vi "Level2a.vi"() -> ()   [LabVIEW 2014]
doc: "Use this template to build a standard state machine design pattern. Each state executes code and determines which state to transition to. Contrast this design pattern with the User Interface Event Handler pattern, in which code executes in response to user actions. Contrast this design pattern also with the Queued Message Handler pattern, in which each message handling code can queue zero or more new messages."
uses:
  subVIs/Level2aState.ctl
panel:
  out "Current Time":timestamp format="%<%I:%M:%S %p\n%x>T"
  out "Input Data":dbl(graph)
  in  "Timer 2 Enabled":bool
  in  "Timer 1 Enabled":bool
  in  "Stop":bool
  out "Value > 0?":bool
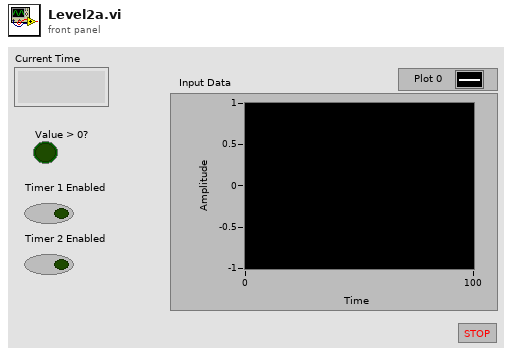
[diagram p1: front panel]
types:
  T1 = typedef "Level2aState.ctl" = enum16{"Check Inputs", "Check Clocks", "Clocks OnOff", "Generate Data", "Update Clock", "Stop"}
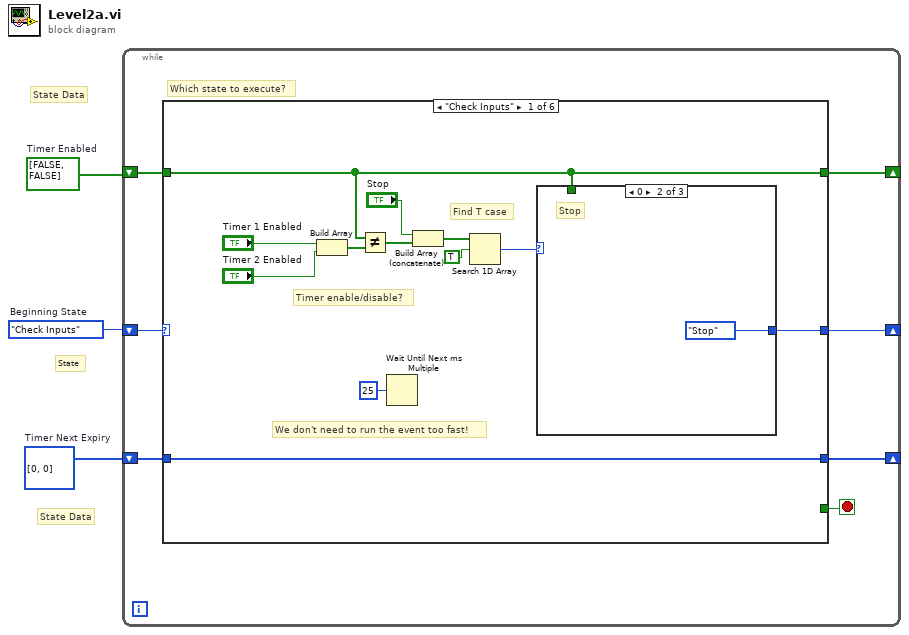
[diagram p0: block diagram]
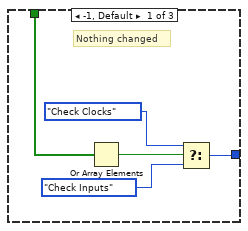
[diagram p2: hidden frame]
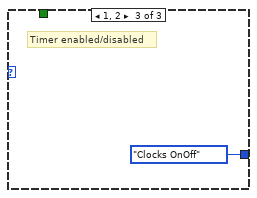
[diagram p3: hidden frame]
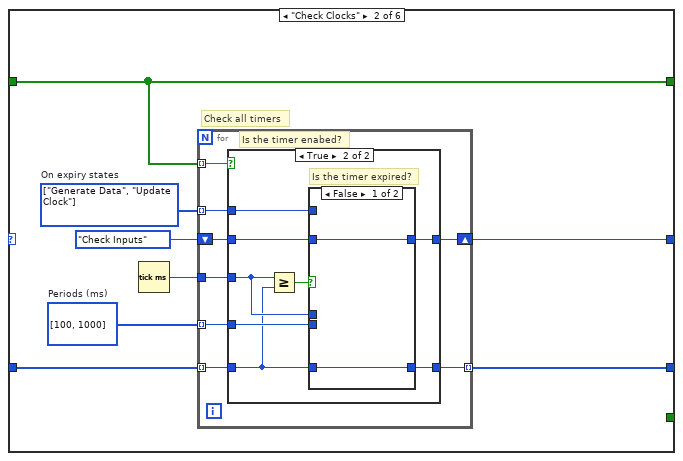
[diagram p4: hidden frame]
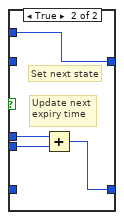
[diagram p6: hidden frame]
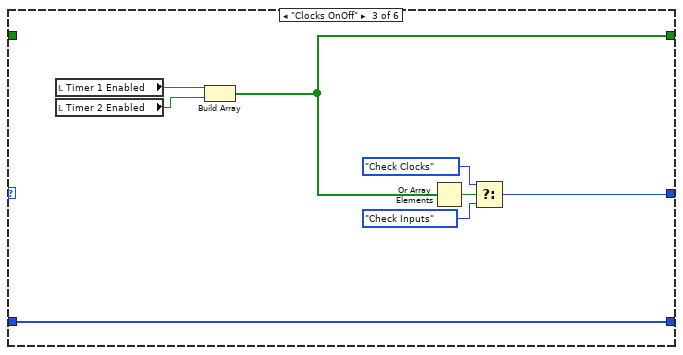
[diagram p7: hidden frame]
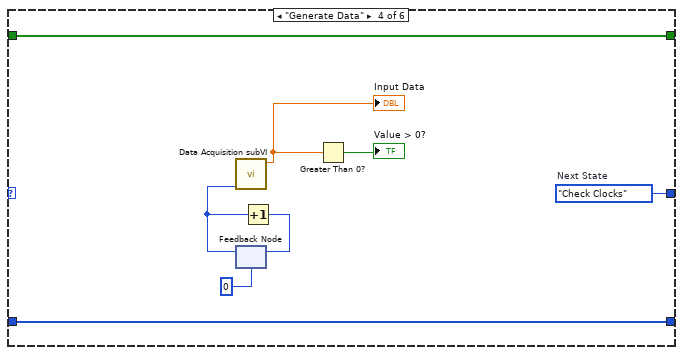
[diagram p8: hidden frame]
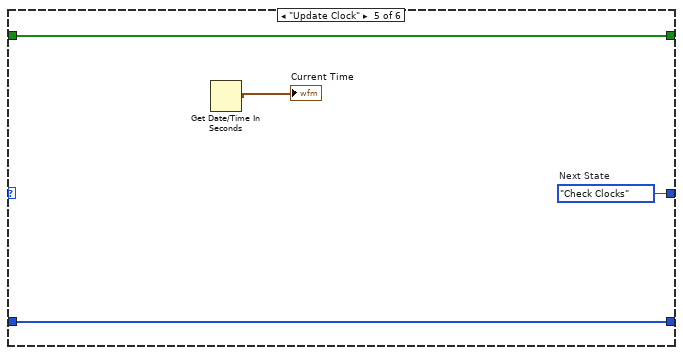
[diagram p9: hidden frame]
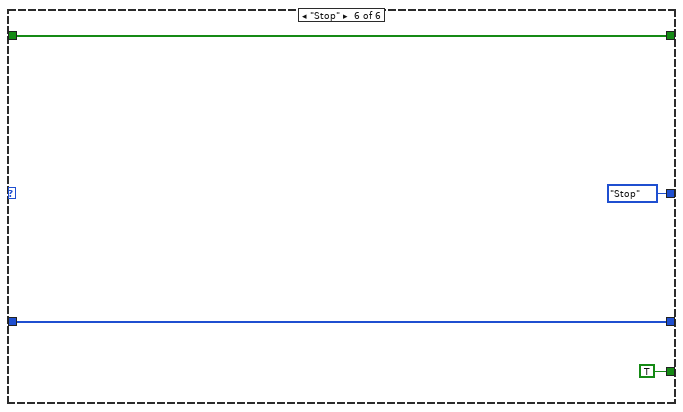
[diagram p10: hidden frame]
diagram:
  w1 = bool[] [FALSE, FALSE]  # Timer Enabled
  w2 = u32[] [0, 0]  # Timer Next Expiry
  w3 = Level2aState."Check Inputs"  # Beginning State
  # "State"
  # "State Data"
  # "State Data"
  n1 = while {
    shift-right: [w6] -> _
    shift-left: w3 -> [w9]
    shift-right: [w5] -> _
    shift-left: w2 -> [w10]
    shift-right: [w7] -> _
    shift-left: w1 -> [w8]
    stop <- w4 stop-if-true
    # "Which state to execute?"
    n2 = case shown="\"Check Inputs\"" w9 {
      tunnel: w10 -> [w12 w37 w62 w75 w80 w83]
      tunnel: w8 -> [w13 w36 _ w77 w81 w82]
      tunnel: [w13 w36 w67 w77 w81 w82] -> w7
      tunnel: [w14 w32 w63 w76 w79 Level2aState."Stop" ("Next State")] -> w6
      tunnel: [w12 w31 w62 w75 w80 w83] -> w5
      tunnel: [_ _ _ _ _ TRUE] -> w4
      frame "Check Inputs" {
        # "We don't need to run the event too fast!"
        # "Find T case"
        # "Timer enable/disable?"
        n3 = Build Array("Timer 1 Enabled", "Timer 2 Enabled") -> (w20:bool[])
        n4 = Not Equal?(x=w13, y=w20) -> (x != y?=w18:bool[])
        n5 = Wait Until Next ms Multiple(millisecond multiple=u32 25) -> ()  [unwired: 1 out]
        n6 = Build Array (concatenate)("Stop", w18) -> (w17:bool[])
        n7 = Search 1D Array(1D array=w17, element=TRUE) -> (index of element=w15:i32)  [unwired: 1 in]
        n8 = case shown="0" w15 {
          tunnel: [w23 Level2aState."Stop" ("States") Level2aState."Clocks OnOff" ("States")] -> w14
          tunnel: w13 -> [w27 _ _]
          frame -1, Default {
            # "Nothing changed"
            n9 = Or Array Elements(Boolean array=w27) -> (logical OR=w26:bool)
            n10 = Select(t=Level2aState."Check Clocks" ("States"), s=w26, f=Level2aState."Check Inputs" ("States")) -> (s? t:f=w23:T1)
          }
          frame 0 {
            # "Stop"
          }
          frame 1, 2 {
            # "Timer enabled/disabled"
          }
        }
      }
      frame "Check Clocks" {
        w33 = T1[] [enum."Generate Data", enum."Update Clock"] items=["Check Inputs", "Check Clocks", "Clocks OnOff", "Generate Data", "Update Clock", "Stop"]  # On expiry states
        w34 = u32[] [100, 1000]  # Periods (ms)
        # "Check all timers"
        n11 = Tick Count (ms)() -> (millisecond timer value=w35:u32)
        n12 = for {
          tunnel: w37 -> [w43] mode=indexing
          tunnel: w36 -> [w45] mode=indexing
          tunnel: [w44] -> w31 mode=indexing
          shift-right: [w38] -> w32
          shift-left: Level2aState."Check Inputs" -> [w42]
          tunnel: w35 -> [w41]
          tunnel: w34 -> [w40] mode=indexing
          tunnel: w33 -> [w39] mode=indexing
          # "Is the timer enabed?"
          n13 = case shown="True" w45 {
            tunnel: [w47 w52] -> w44
            tunnel: w43 -> [w47 w51]
            tunnel: w42 -> [w46 w48]
            tunnel: w41 -> [_ w54]
            tunnel: w40 -> [_ w53]
            tunnel: w39 -> [_ w49]
            tunnel: [w46 w50] -> w38
            frame False {
              # "Timer disabled"
            }
            frame True {
              # "Is the timer expired?"
              n14 = Greater Or Equal?(x=w54, y=w51) -> (x >= y?=w55:bool)
              n15 = case shown="False" w55 {
                tunnel: w54 -> [_ w61]
                tunnel: w53 -> [_ w60]
                tunnel: [w57 w59] -> w52
                tunnel: w51 -> [w57 _]
                tunnel: [w56 w58] -> w50
                tunnel: w49 -> [_ w58]
                tunnel: w48 -> [w56 _]
                frame False {
                }
                frame True {
                  # "Set next state"
                  # "Update next\nexpiry time"
                  n16 = Add(x=w61, y=w60) -> (x+y=w59:u32)
                }
              }
            }
          }
        }
      }
      frame "Clocks OnOff" {
        n17 = local read "Timer 1 Enabled"() -> (w69:bool)
        n18 = local read "Timer 2 Enabled"() -> (w68:bool)
        n19 = Build Array(w69, w68) -> (w67:bool[])
        n20 = Or Array Elements(Boolean array=w67) -> (logical OR=w66:bool)
        n21 = Select(t=Level2aState."Check Clocks" ("Beginning State"), s=w66, f=Level2aState."Check Inputs" ("Beginning State")) -> (s? t:f=w63:T1)
      }
      frame "Generate Data" {
        w76 = Level2aState."Check Clocks"  # Next State
        n22 = feedback #1(0) -> (w72:i32)
        n23 = call "Data Acquisition subVI.vi"("Numeric in"=w72) -> ("Numeric out"=w71:dbl)  [unwired: 10 in]
        "Input Data" <- w71
        n24 = Increment(x=w72) -> (x+1=w74:i32)
        n25 = feedback-in #1(w74) -> ()
        n26 = Greater Than 0?(x=w71) -> (x > 0?=→"Value > 0?":bool)
      }
      frame "Update Clock" {
        w79 = Level2aState."Check Clocks"  # Next State
        n27 = Get Date/Time In Seconds() -> (seconds since 1Jan1904=→"Current Time":timestamp)
      }
      frame "Stop" {
      }
    }
  }
